vi "DIO64 CheckOS.vi"(8 "error in":errorcluster) -> (0 "error out":errorcluster, 3 "path in":path=path "DIO64_Visa32.dll")   [LabVIEW 2012]
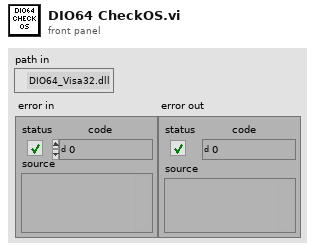
[diagram p1: front panel]
types:
  T1 = enum32{"invalid OS target", "Mac OS", "Windows 3.1", "Windows 95/NT", "Solaris 1", "Solaris 2", "HP-UX", "PowerMAX", "Linux", "Irix", "Rhapsody", "BeOS", "AIX", "OSF1", "VxWorks", "PharLap", "Carbon", "RTX", "Windows x64", "Linux x64"}
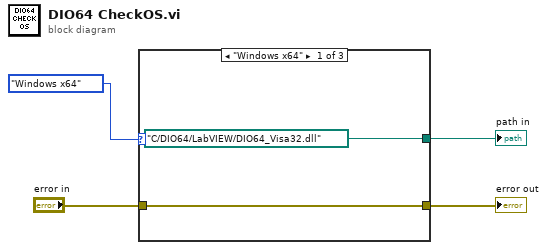
[diagram p0: block diagram]
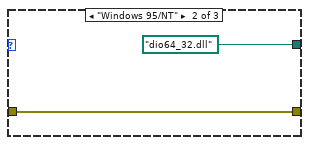
[diagram p2: hidden frame]
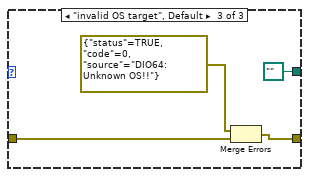
[diagram p3: hidden frame]
diagram:
  n1 = case shown="\"Windows x64\"" T1."Windows x64" ("Application:Target:Operating System") {
    tunnel: [path "C:/DIO64/LabVIEW/DIO64_Visa32.dll" ("path in") path "dio64_32.dll" ("path in") path "" ("path in")] -> w4
    tunnel: [w5 w7 w10] -> w3
    tunnel: "error in" -> [w5 w7 w11]
    frame "Windows x64" {
    }
    frame "Windows 95/NT" {
    }
    frame "invalid OS target", Default {
      n2 = Merge Errors(errorcluster {"status"=TRUE, "code"=0, "source"="DIO64: Unknown OS!!"} ("error constant"), w11) -> (w10:errorcluster)
    }
  }
  "path in" <- w4
  "error out" <- w3
